vi "Read Attributes.vi"(11 "Island Microgrid Msg":refnum<class "Island Microgrid Msg.lvclass">) -> (2 "Payload":cluster{"Data":variant})   [LabVIEW 2018, in "Remote Operation Abstract.lvlib" / "Island Microgrid Msg.lvclass"]
uses:
  Island Microgrid Msg.lvclass
  Island Microgrid Msg.lvclass/Island Microgrid Msg.ctl
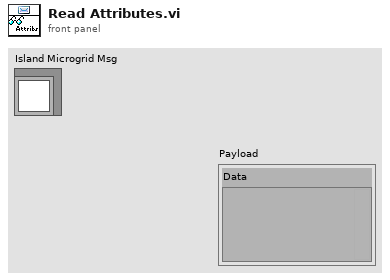
[diagram p1: front panel]
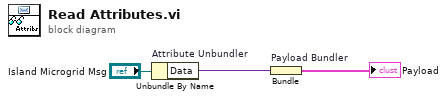
[diagram p0: block diagram]
diagram:
  n1 = Unbundle By Name "Attribute Unbundler"("Island Microgrid Msg") -> ("Data"=w1:variant)
  n2 = Bundle "Payload Bundler"("Data"=w1) -> (→"Payload":cluster{"Data":variant})  [unwired: 1 in]
